vi "21414111邱致綸.vi"() -> ()   [LabVIEW 2017]
panel:
  out "交大":bool
  out "台大":bool
  out "成大":bool
  out "落榜":bool
  in  "數學":bool
  in  "理化":bool
  in  "英文":bool
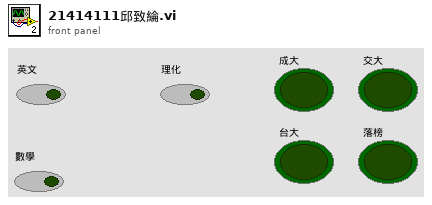
[diagram p1: front panel]
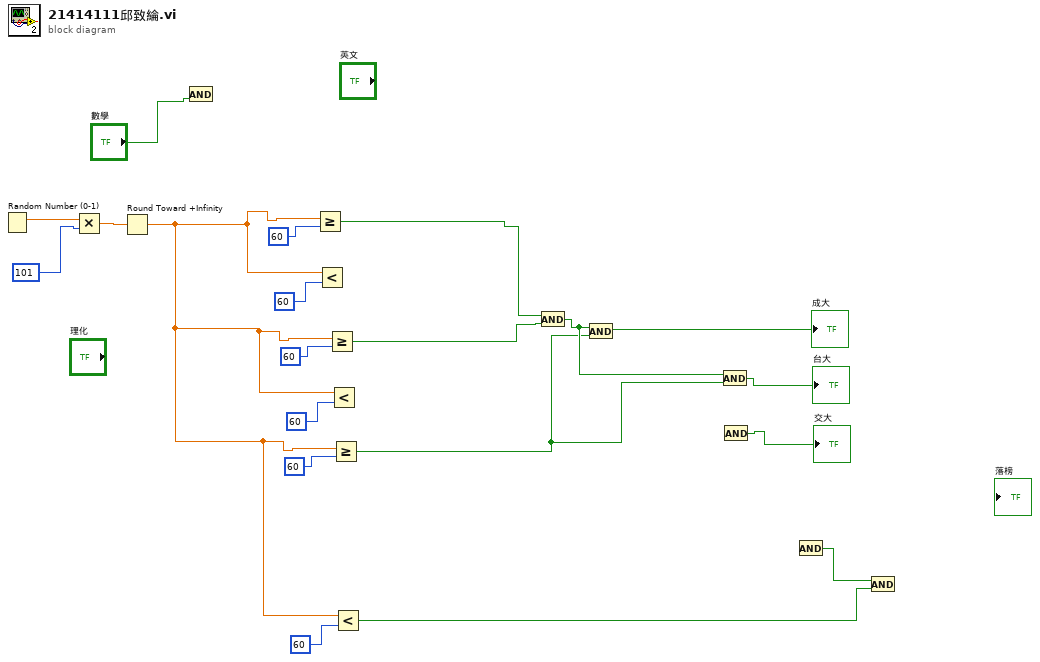
[diagram p0: block diagram]
diagram:
  n1 = Random Number (0-1)() -> (number: 0 to 1=w19:dbl)
  n2 = Multiply(x=w19, y=101) -> (x*y=w17:dbl)
  n3 = Round Toward +Infinity(x=w17) -> (ceil(x): smallest int >= x=w7:dbl)
  n4 = And(y="數學") -> ()  [unwired: 1 in, 1 out]
  n5 = Greater Or Equal?(x=w7, y=60) -> (x >= y?=w14:bool)
  n6 = Less?(x=w7, y=60) -> ()  [unwired: 1 out]
  n7 = Greater Or Equal?(x=w7, y=60) -> (x >= y?=w11:bool)
  n8 = Less?(x=w7, y=60) -> ()  [unwired: 1 out]
  n9 = Greater Or Equal?(x=w7, y=60) -> (x >= y?=w3:bool)
  n10 = Less?(x=w7, y=60) -> (x < y?=w6:bool)
  n11 = And(x=w14, y=w11) -> (x .and. y?=w4:bool)
  n12 = And(x=w4, y=w3) -> (x .and. y?=→"成大":bool)
  n13 = And(x=w4, y=w3) -> (x .and. y?=→"台大":bool)
  n14 = And() -> (x .and. y?=→"交大":bool)  [unwired: 2 in]
  n15 = And() -> (x .and. y?=w10:bool)  [unwired: 2 in]
  n16 = And(x=w10, y=w6) -> ()  [unwired: 1 out]
